vi "Packet Size Benchmark Test App.vi"() -> ()   [LabVIEW 2011]
uses:
  <vilib>/Instr/_visa.llb/VISA Configure Serial Port (Instr).vi
  <vilib>/ptbypt/NI_PtbyPt.lvlib
panel:
  out "Graph 2":cluster{i32, u32}[](graph)
  out "Progress Bar":u8(slide) scale=0.0..100.0
  out "Graph":T1(graph)
  out "Average Loop Time":u32
  out "Min Loop Time (ms)":u32
  out "Max Loop Time (ms)":u32
  out "Failed Packets":u32
  in  "# Packets To Send":i32=256
  in  "Packet Size":u8=3
  in  "COM Port":refnum<visa-resource-name>="COM4"
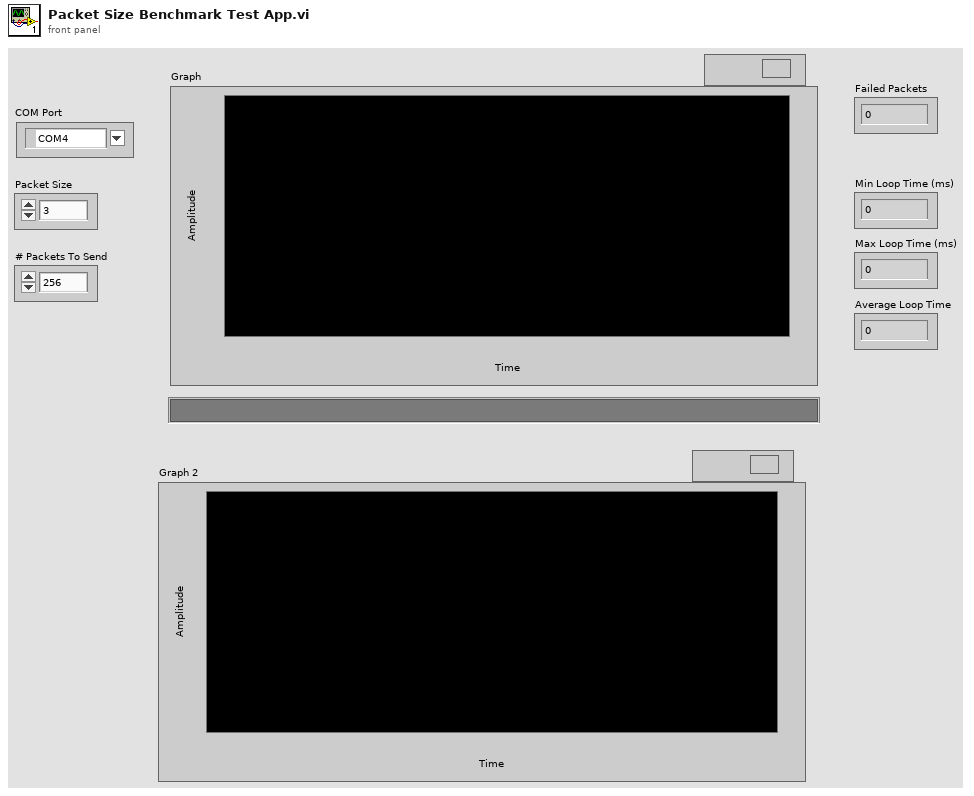
[diagram p1: front panel]
types:
  T1 = cluster{"X Values":dbl[], "Histogram: h(x)":i32[]}
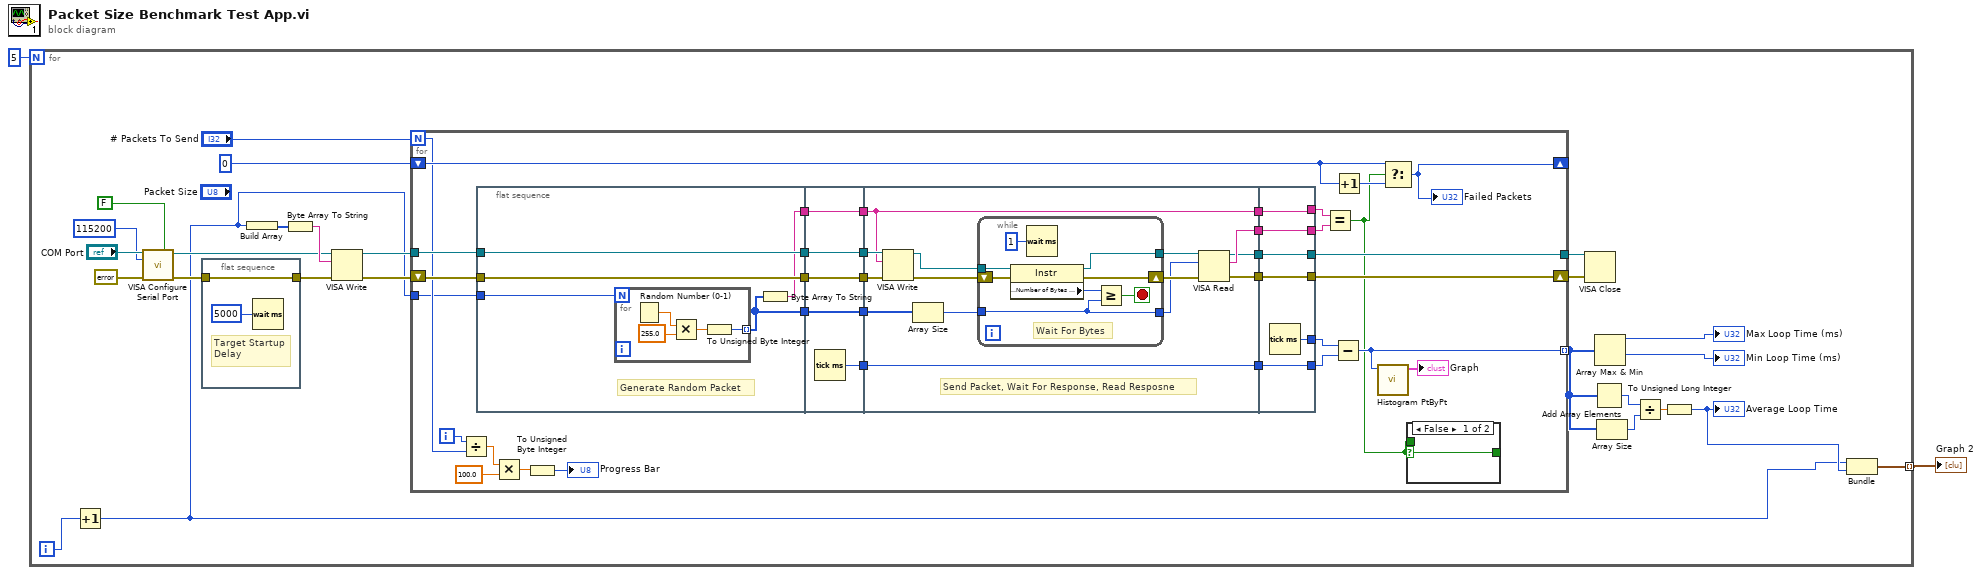
[diagram p0: block diagram]
diagram:
  n1 = for {
    N: 5 -> [_]
    tunnel: [w5] -> w1 mode=indexing
    i -> [w6]
    n2 = Increment(x=w6) -> (x+1=w3:i32)
    n3 = call-poly "VISA Configure Serial Port"("VISA resource name"="COM Port", "Enable Termination\nChar (T)"=FALSE ("Enable Termination\nChar (T)"), "baud rate (9600)"=u32 115200, "error in (no error)"=errorcluster {"status"=FALSE, "code"=0, "source"=""}) -> ("VISA resource name out"=w8:refnum<visa-resource-name>, "error out"=w24:errorcluster)  [unwired: 10 in]
    n4 = flat-sequence {
      tunnel: [w28] -> w13
      tunnel: w24 -> [w28]
      frame #0 {
        # "Target Startup\nDelay"
        n5 = Wait (ms)(milliseconds to wait=u32 5000) -> ()  [unwired: 1 out]
      }
    }
    n6 = Build Array(w3) -> (w12:i32[])
    n7 = Byte Array To String(unsigned byte array=w12) -> (string=w11:string)
    n8 = VISA Write(VISA resource name=w8, write buffer=w11, error in (no error)=w13) -> (VISA resource name out=w10:refnum<visa-resource-name>, error out=w9:errorcluster)  [unwired: 1 out]
    n9 = for {
      N: "# Packets To Send" -> [w40]
      tunnel: w10 -> [w50]
      tunnel: [w48] -> w16
      tunnel: [w42] -> w20 mode=indexing
      shift-right: [w33] -> _
      shift-left: u32 0 ("baud rate (9600)") -> [w44]
      shift-right: [w49] -> w15
      shift-left: w9 -> [w43]
      tunnel: w3 -> [w34]
      i -> [w38]
      n10 = Divide(x=w38, y=w40) -> (x/y=w37:dbl)
      n11 = flat-sequence {
        tunnel: [w71] -> w64
        tunnel: [w70] -> w63
        tunnel: [w69] -> w62
        tunnel: [w68] -> w61
        tunnel: w50 -> [w71]
        tunnel: w43 -> [w70]
        tunnel: w34 -> [w67]
        tunnel: [w80] -> w60
        tunnel: [w79] -> w59
        tunnel: [w78] -> w58
        tunnel: w64 -> [w80]
        tunnel: w63 -> [w79]
        tunnel: [w77] -> w57
        tunnel: w62 -> [w77]
        tunnel: [w76] -> w56
        tunnel: w61 -> [w76]
        tunnel: w60 -> [w94]
        tunnel: w59 -> [w93]
        tunnel: [w87] -> w55
        tunnel: [w86] -> w54
        tunnel: [w81] -> w53
        tunnel: w58 -> [w85]
        tunnel: [w85] -> w52
        tunnel: w57 -> [w84]
        tunnel: w56 -> [w83]
        tunnel: [w83] -> w51
        tunnel: [w106] -> w48
        tunnel: [w107] -> w49
        tunnel: [w108] -> w31
        tunnel: w55 -> [w108]
        tunnel: w54 -> [w107]
        tunnel: w53 -> [w106]
        tunnel: [w105] -> w47
        tunnel: w52 -> [w104]
        tunnel: [w104] -> w46
        tunnel: w51 -> [w103]
        tunnel: [w103] -> w32
        frame #0 {
          # "Generate Random Packet"
          n12 = for {
            N: w67 -> [_]
            tunnel: [w72] -> w69 mode=indexing
            n13 = Random Number (0-1)() -> (number: 0 to 1=w75:dbl)
            n14 = Multiply(x=w75, y=255.0) -> (x*y=w73:dbl)
            n15 = To Unsigned Byte Integer(number=w73) -> (unsigned 8bit integer=w72:u8)
          }
          n16 = Byte Array To String(unsigned byte array=w69) -> (string=w68:string)
        }
        frame #1 {
          n17 = Tick Count (ms)() -> (millisecond timer value=w78:u32)
        }
        frame #2 {
          # "Send Packet, Wait For Response, Read Resposne"
          n18 = VISA Write(VISA resource name=w94, write buffer=w83, error in (no error)=w93) -> (VISA resource name out=w92:refnum<visa-resource-name>, error out=w91:errorcluster)  [unwired: 1 out]
          n19 = Array Size(array=w84) -> (size(s)=w90:i32)
          n20 = while "Wait For Bytes" {
            tunnel: w92 -> [w102]
            tunnel: w90 -> [w96]
            shift-right: [w100] -> w89
            shift-left: w91 -> [w101]
            tunnel: [w99] -> w88
            tunnel: [w96] -> w82
            stop <- w97 stop-if-true
            # "Wait For Bytes"
            n21 = property class="Instr"(reference=w102, error in=w101) -> (reference out=w99:refnum<visa-resource-name>, error out=w100:errorcluster, "Serial Settings:Number of Bytes at Serial Port"=w98:u32)
            n22 = Wait (ms)(milliseconds to wait=u32 1) -> ()  [unwired: 1 out]
            n23 = Greater Or Equal?(x=w98, y=w96) -> (x >= y?=w97:bool)
          }
          n24 = VISA Read(VISA resource name=w88, byte count=w82, error in (no error)=w89) -> (VISA resource name out=w81:refnum<visa-resource-name>, read buffer=w87:string, error out=w86:errorcluster)  [unwired: 1 out]
        }
        frame #3 {
          n25 = Tick Count (ms)() -> (millisecond timer value=w105:u32)
        }
      }
      n26 = Multiply(x=w37, y=100.0) -> (x*y=w35:dbl)
      n27 = To Unsigned Byte Integer(number=w35) -> (unsigned 8bit integer=→"Progress Bar":u8)
      n28 = Equal?(x=w32, y=w31) -> (x = y?=w30:bool)
      n29 = Subtract(x=w47, y=w46) -> (x-y=w42:u32)
      n30 = Increment(x=w44) -> (x+1=w45:u32)
      n31 = call <vilib>:"Histogram PtByPt.vi"("x"=w42) -> ("Histogram Graph"=→"Graph":T1)  [unwired: 7 in, 3 out]
      n32 = Select(t=w44, s=w30, f=w45) -> (s? t:f=w33:u32)
      "Failed Packets" <- w33
      n33 = case shown="False" w30 {
        selector: w30 -> [w65 _]
        tunnel: [w65 w66] -> _
        tunnel: w30 -> [_ w66]
        frame False {
        }
        frame True {
        }
      }
    }
    n34 = VISA Close(VISA resource name=w16, error in (no error)=w15) -> ()  [unwired: 1 out]
    n35 = Add Array Elements(numeric array=w20) -> (sum=w21:u32)
    n36 = Array Max & Min(array=w20) -> (max value=→"Max Loop Time (ms)":u32, min value=→"Min Loop Time (ms)":u32)  [unwired: 2 out]
    n37 = Array Size(array=w20) -> (size(s)=w19:i32)
    n38 = Divide(x=w21, y=w19) -> (x/y=w14:dbl)
    n39 = To Unsigned Long Integer(number=w14) -> (unsigned 32bit integer=w4:u32)
    "Average Loop Time" <- w4
    n40 = Bundle(w3, w4) -> (w5:cluster{i32, u32})  [unwired: 1 in]
  }
  "Graph 2" <- w1
